vi "Create Queue.vi"(8 "error in":errorcluster, 11 "Process Name":string) -> (0 "error out":errorcluster, 3 "queue out":refnum<queue>)   [LabVIEW 2020, in "Internal Messaging Library.lvlib"]
uses:
  Internal Messaging Library.lvlib
  Controls/Messaging Cluster.ctl
  Controls/Message.ctl
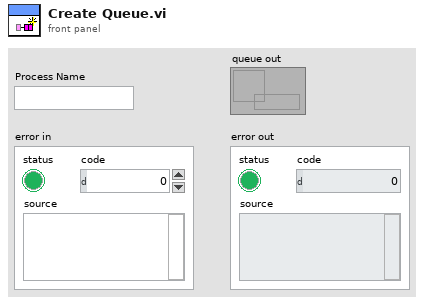
[diagram p1: front panel]
types:
  T1 = typedef "Internal Messaging Library.lvlib/Messaging Cluster.ctl" = cluster{"Message":T2, "Data":variant}
  T2 = typedef "Internal Messaging Library.lvlib/Message.ctl" = enum16{"Initialize", "Exit", "Error", "Load Data", "Add Time Entry", "Modify Time Entry", "Delete Time Entry"}
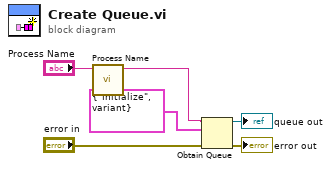
[diagram p0: block diagram]
diagram:
  n1 = call "Process Name.vi"("Process Name"="Process Name") -> ("Process Name"=w5:string)  [unwired: 10 in]
  n2 = Obtain Queue(name (unnamed)=w5, element data type=T1 {"Message"=enum."Initialize", "Data"=variant} ("Messaging Cluster"), error in (no error)="error in") -> (queue out=→"queue out":refnum<queue>, error out=→"error out":errorcluster)  [unwired: 2 in, 1 out]
